vi "Test Loop.vi"() -> ()   [LabVIEW 2023]
panel:
  in  "stop":bool
  out "Loop Index":i32
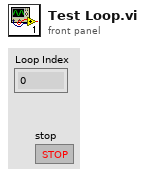
[diagram p1: front panel]
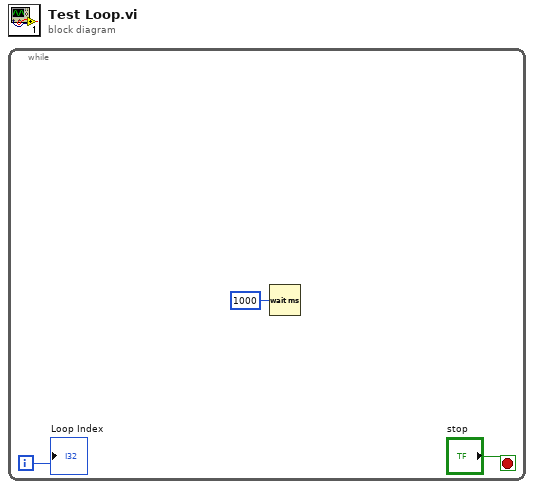
[diagram p0: block diagram]
diagram:
  n1 = while {
    i -> [w3]
    stop <- "stop" stop-if-true
    n2 = Wait (ms)(milliseconds to wait=u32 1000) -> ()  [unwired: 1 out]
    "Loop Index" <- w3
  }
